vi "UpdateVoltResultFixture_1.vi"(7 "Auto FL/FR":bool, 8 "Test Name":string(combo)="Door Lock", 9 "Result 2":bool=TRUE, 10 "Result 1":bool=TRUE, 11 "Fixture Array Input":u16[](array[numeric])) -> (0 "Result":bool, 3 "Fixture Array Output":u16[](array[numeric]))   [LabVIEW 2017]
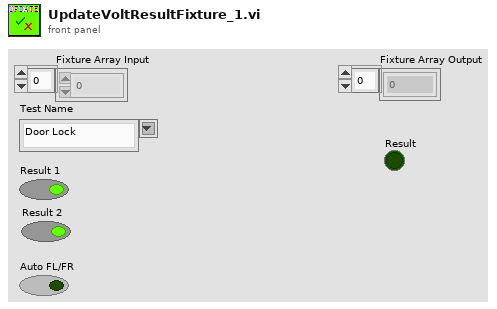
[diagram p1: front panel]
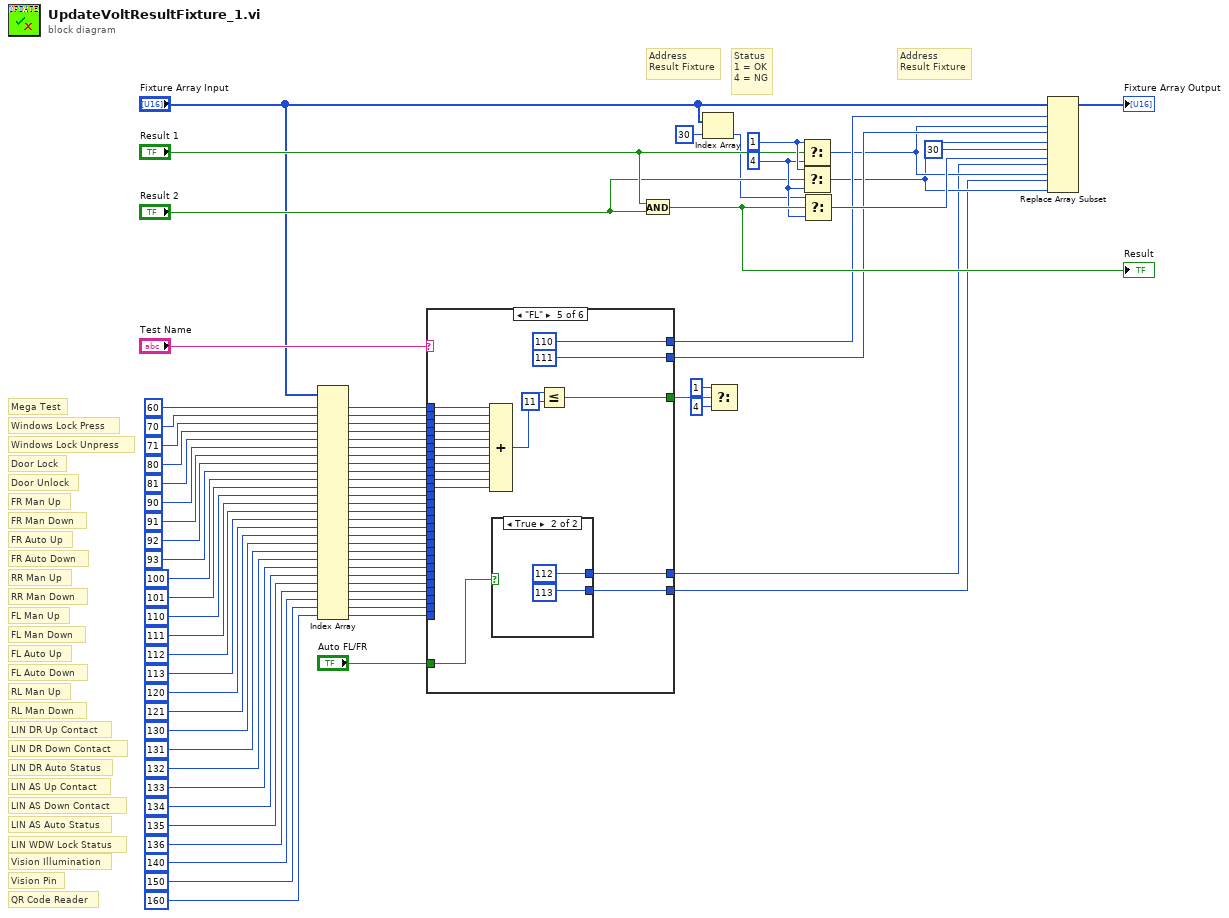
[diagram p0: block diagram]
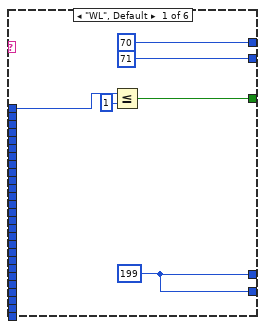
[diagram p2: hidden frame]
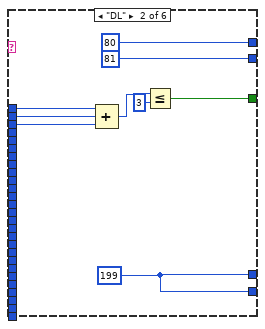
[diagram p3: hidden frame]
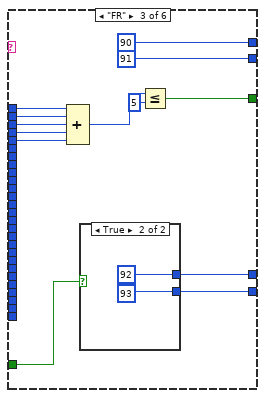
[diagram p4: hidden frame]
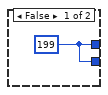
[diagram p5: hidden frame]
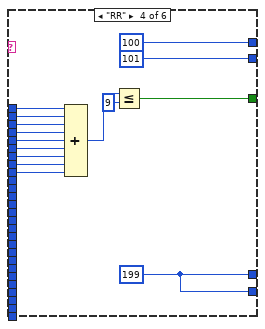
[diagram p6: hidden frame]
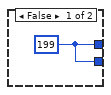
[diagram p7: hidden frame]
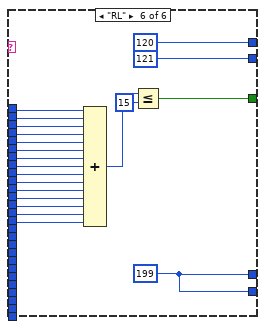
[diagram p8: hidden frame]
diagram:
  w73 = 4
  w76 = 1
  # "Address\nResult Fixture"
  # "Status\n1 = OK\n4 = NG"
  # "Address\nResult Fixture"
  # "LIN WDW Lock Status"
  # "QR Code Reader"
  # "Vision Pin"
  # "Vision Illumination"
  # "LIN AS Auto Status"
  # "LIN AS Down Contact"
  # "LIN AS Up Contact"
  # "LIN DR Auto Status"
  # "LIN DR Down Contact"
  # "LIN DR Up Contact"
  # "RL Man Down"
  # "RL Man Up"
  # "FL Auto Down"
  # "FL Auto Up"
  # "FL Man Down"
  # "FL Man Up"
  # "RR Man Down"
  # "RR Man Up"
  # "FR Auto Down"
  # "FR Auto Up"
  # "FR Man Down"
  # "FR Man Up"
  # "Door Unlock"
  # "Door Lock"
  # "Windows Lock Unpress"
  # "Windows Lock Press"
  # "Mega Test"
  n1 = Index Array(array="Fixture Array Input", index #1=60 ("index"), index #2=70 ("index"), index #3=71 ("index"), index #4=80 ("index"), index #5=81 ("index"), index #6=90 ("index"), index #7=91 ("index"), index #8=92 ("index"), index #9=93 ("index"), index #10=100 ("index"), index #11=101 ("index"), index #12=110 ("index"), index #13=111 ("index"), index #14=112 ("index"), index #15=113 ("index"), index #16=120 ("index"), index #17=121 ("index"), index #18=130 ("index"), index #19=131 ("index"), index #20=132 ("index"), index #21=133 ("index"), index #22=134 ("index"), index #23=135 ("index"), index #24=136 ("index"), index #25=140 ("index"), index #26=150 ("index"), index #27=160 ("index")) -> (element #1=w36:u16, element #2=w35:u16, element #3=w34:u16, element #4=w33:u16, element #5=w32:u16, element #6=w31:u16, element #7=w30:u16, element #8=w29:u16, element #9=w28:u16, element #10=w27:u16, element #11=w26:u16, element #12=w25:u16, element #13=w24:u16, element #14=w23:u16, element #15=w22:u16, element #16=w21:u16, element #17=w20:u16, element #18=w19:u16, element #19=w18:u16, element #20=w17:u16, element #21=w16:u16, element #22=w15:u16, element #23=w14:u16, element #24=w13:u16, element #25=w12:u16, element #26=w11:u16, element #27=w10:u16)
  n2 = case shown="\"FL\"" "Test Name" {
    tunnel: [70 ("index") 80 ("index") 90 ("index") 100 ("index") 110 ("index") 120 ("index")] -> w67
    tunnel: [71 ("index") 81 ("index") 91 ("index") 101 ("index") 111 ("index") 121 ("index")] -> w66
    tunnel: w36 -> [w80 w89 w100 w118 w137 w161]
    tunnel: w35 -> [_ w88 w98 w116 w136 w160]
    tunnel: w34 -> [_ w87 w97 w115 w135 w159]
    tunnel: w33 -> [_ _ w96 w114 w133 w158]
    tunnel: w32 -> [_ _ w95 w113 w134 w157]
    tunnel: w31 -> [_ _ _ w112 w132 w156]
    tunnel: w30 -> [_ _ _ w111 w131 w155]
    tunnel: w29 -> [_ _ _ w110 w130 w154]
    tunnel: w28 -> [_ _ _ w109 w129 w153]
    tunnel: w27 -> [_ _ _ _ w128 w152]
    tunnel: w26 -> [_ _ _ _ w127 w151]
    tunnel: w25 -> [_ _ _ _ _ w149]
    tunnel: w24 -> [_ _ _ _ _ w148]
    tunnel: w23 -> [_ _ _ _ _ w146]
    tunnel: w22 -> [_ _ _ _ _ w147]
    tunnel: w21 -> [_ _ _ _ _ _]
    tunnel: w20 -> [_ _ _ _ _ _]
    tunnel: w19 -> [_ _ _ _ _ _]
    tunnel: w18 -> [_ _ _ _ _ _]
    tunnel: w17 -> [_ _ _ _ _ _]
    tunnel: w16 -> [_ _ _ _ _ _]
    tunnel: w15 -> [_ _ _ _ _ _]
    tunnel: w14 -> [_ _ _ _ _ _]
    tunnel: w13 -> [_ _ _ _ _ _]
    tunnel: w12 -> [_ _ _ _ _ _]
    tunnel: w11 -> [_ _ _ _ _ _]
    tunnel: w10 -> [_ _ _ _ _ _]
    tunnel: [w78 w84 w99 w117 w126 w150] -> w8
    tunnel: [w77 w83 w94 w108 w125 w145] -> w4
    tunnel: [w77 w83 w93 w108 w124 w145] -> w3
    tunnel: "Auto FL/FR" -> [_ _ w92 _ w123 _]
    frame "WL", Default {
      w77 = 199 ("index")
      n3 = Less Or Equal?(x=w80, y=u16 1) -> (x <= y?=w78:bool)
    }
    frame "DL" {
      w83 = 199 ("index")
      n4 = Compound Arithmetic op=ADD(w89, w88, w87) -> (w85:u16)
      n5 = Less Or Equal?(x=w85, y=u16 3) -> (x <= y?=w84:bool)
    }
    frame "FR" {
      n6 = Compound Arithmetic op=ADD(w100, w98, w97, w96, w95) -> (w102:u16)
      n7 = case shown="True" w92 {
        tunnel: [w105 92 ("index")] -> w94
        tunnel: [w105 93 ("index")] -> w93
        frame False {
          w105 = 199 ("index")
        }
        frame True {
        }
      }
      n8 = Less Or Equal?(x=w102, y=u16 5) -> (x <= y?=w99:bool)
    }
    frame "RR" {
      w108 = 199 ("index")
      n9 = Compound Arithmetic op=ADD(w118, w116, w115, w114, w113, w112, w111, w110, w109) -> (w120:u16)
      n10 = Less Or Equal?(x=w120, y=u16 9) -> (x <= y?=w117:bool)
    }
    frame "FL" {
      n11 = Compound Arithmetic op=ADD(w137, w136, w135, w133, w134, w132, w131, w130, w129, w128, w127) -> (w139:u16)
      n12 = case shown="True" w123 {
        tunnel: [w142 112 ("index")] -> w125
        tunnel: [w142 113 ("index")] -> w124
        frame False {
          w142 = 199 ("index")
        }
        frame True {
        }
      }
      n13 = Less Or Equal?(x=w139, y=u16 11) -> (x <= y?=w126:bool)
    }
    frame "RL" {
      w145 = 199 ("index")
      n14 = Compound Arithmetic op=ADD(w161, w160, w159, w158, w157, w156, w155, w154, w153, w152, w151, w149, w148, w146, w147) -> (w163:u16)
      n15 = Less Or Equal?(x=w163, y=u16 15) -> (x <= y?=w150:bool)
    }
  }
  n16 = And(x="Result 1", y="Result 2") -> (x .and. y?=w74:bool)
  "Result" <- w74
  n17 = Index Array(array="Fixture Array Input", index=30) -> (element=w1:u16)
  n18 = Select(t=1, s=w8, f=4) -> ()  [unwired: 1 out]
  n19 = Select(t=w76, s="Result 1", f=w73) -> (s? t:f=w6:i32)
  n20 = Select(t=w76, s="Result 2", f=w73) -> (s? t:f=w5:i32)
  n21 = Select(t=w1, s=w74, f=w73) -> (s? t:f=w71:i32)
  n22 = Replace Array Subset(array="Fixture Array Input", new element #1=w6, index #1=w67, new element #2=w5, index #2=w66, new element #3=w71, index #3=30 ("index"), new element #4=w6, index #4=w4, new element #5=w5, index #5=w3) -> (→"Fixture Array Output":u16[])
